vi "dfd_BW Lowpass S Poles and Zeros.vi"(2 "low cutoff freq: wl":dbl=0.125 format="%.3f", 3 "order":i32=2) -> (0 "zeros":T1[](array[typedef]), 1 "poles":T1[](array[typedef]))   [LabVIEW 2017, in "NI_DigFilter_Design.lvlib"]
uses:
  <vilib>/addons/Digital Filter Design/NI_DigFilter_Design.lvlib
  <vilib>/addons/Digital Filter Design/_Objects.llb/DFD Pole-Zero.ctl
  <vilib>/addons/Digital Filter Design/NI_DigFilterLicensed.lvlib
panel:
  in  "DFD Zero Pole":T1={"value"=0.0+0.0i, "z attr"={"real"=FALSE, "lp"=FALSE, "uc"=FALSE}, "order"=1}
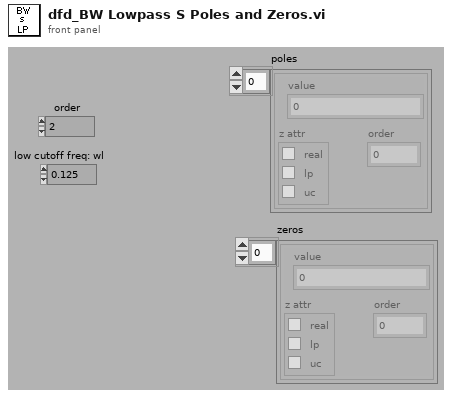
[diagram p1: front panel]
types:
  T1 = typedef "NI_DigFilterLicensed.lvlib/DFD Pole-Zero.ctl" = cluster{"value":cdb, "z attr":cluster{"real":bool, "lp":bool, "uc":bool}, "order":i32}
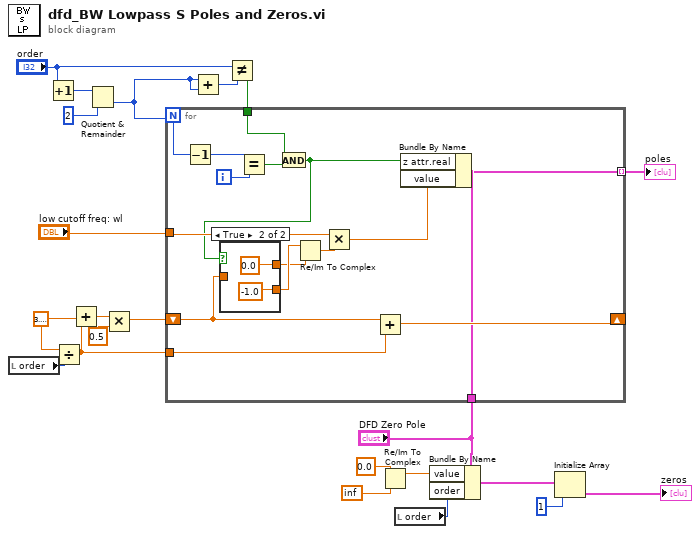
[diagram p0: block diagram]
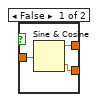
[diagram p2: hidden frame]
diagram:
  w8 = 3.141592653589793
  n1 = local read "order"() -> (w21:i32)
  n2 = Increment(x="order") -> (x+1=w16:i32)
  n3 = Divide(x=w8, y=w21) -> (x/y=w20:dbl)
  n4 = Add(x=w8, y=w20) -> (x+y=w18:dbl)
  n5 = Quotient & Remainder(x=w16, y=2) -> (floor(x/y)=w1:i32)  [unwired: 1 out]
  n6 = Multiply(x=w18, y=0.5) -> (x*y=w17:dbl)
  n7 = Add(x=w1, y=w1) -> (x+y=w13:i32)
  n8 = Not Equal?(x="order", y=w13) -> (x != y?=w12:bool)
  n9 = for {
    N: w1 -> [w32]
    shift-right: [w37] -> _
    shift-left: w17 -> [w24]
    tunnel: w20 -> [w38]
    tunnel: "low cutoff freq: wl" -> [w35]
    tunnel: "DFD Zero Pole" -> [w30]
    tunnel: [w29] -> w14 mode=indexing
    tunnel: w12 -> [w23]
    i -> [w34]
    n10 = Decrement(x=w32) -> (x-1=w33:i32)
    n11 = Equal?(x=w33, y=w34) -> (x = y?=w31:bool)
    n12 = And(x=w23, y=w31) -> (x .and. y?=w25:bool)
    n13 = case shown="True" w25 {
      tunnel: w24 -> [w41 _]
      tunnel: [w40 -1.0] -> w27
      tunnel: [w39 0.0] -> w26
      frame False {
        n14 = Sine & Cosine(0:w41) -> (1:w39:dbl, 2:w40:dbl)
      }
      frame True {
      }
    }
    n15 = Re/Im To Complex(1:w26, 2:w27) -> (0:w36:cdb)
    n16 = Multiply(x=w35, y=w36) -> (x*y=w28:cdb)
    n17 = Add(x=w24, y=w38) -> (x+y=w37:dbl)
    n18 = Bundle By Name(cluster=w30, "z attr.real"=w25, "value"=w28) -> (w29:T1)
  }
  "poles" <- w14
  n19 = Re/Im To Complex(1:inf, 2:0.0) -> (0:w5:cdb)
  n20 = local read "order"() -> (w10:i32)
  n21 = Bundle By Name(cluster="DFD Zero Pole", "value"=w5, "order"=w10) -> (w11:T1)
  n22 = Initialize Array(w11, 1) -> (→"zeros":T1[])
